vi "Lab Panel V6.00.vi"() -> ()   [LabVIEW 2017] (continued)
                    n3246 = call "sub vi-open serial port v1.vi"("Select COM port"=w5964) -> ("Error"=w5963:bool, "LOOPS"=w5962:i32, "VISA Com out"=w5961:refnum<visa-resource-name>)  [unwired: 12 in]
                    n3247 = local write "Com setup loops"(w5962) -> ()
                    n3248 = local write "Com Port Status"(w5963) -> ()
                    n3249 = local write "VISA Com out"(w5961) -> ()
                    n3250 = global write "Global 1.vi" "COM port"(w5961) -> ()
                  }
                }
              }
              frame #1 {
                # "only get temperature from initial valid temperature circuits, circuits detected at startup time"
                n3251 = local read "VISA Com out"() -> (w5974:refnum<visa-resource-name>)
                n3252 = global write "Global 1.vi" "COM port"(w5974) -> ()
                n3253 = local read "Temp read loop"() -> (w5971:dbl)
                n3254 = global write "Global 1.vi" "tmp dly lps"("Temp Delay Lps") -> ()
                n3255 = global write "Global 1.vi" "dly value"("Temp Value") -> ()
                n3256 = local read "jig cycle"() -> (w5975:dbl)
                n3257 = local read "on loops"() -> (w5977:dbl)
                n3258 = Equal?(x=w5971, y=1) -> (x = y?=w5968:bool)
                n3259 = Add(x=w5977, y=6) -> (x+y=w5978:dbl)
                n3260 = Equal?(x=w5975, y=w5978) -> (x = y?=w5969:bool)
                n3261 = And(x=w5969, y=w5968) -> (x .and. y?=w5967:bool)
                n3262 = Or(x=w5967, y="Read Temp") -> (x .or. y?=w5966:bool)
                n3263 = case shown="True" w5966 {
                  frame False {
                  }
                  frame True {
                    w5979 = TRUE
                    n3264 = local write "TEMP"(w5979) -> ()
                    n3265 = local write "Read Temp"(FALSE) -> ()
                    n3266 = stacked-sequence {
                      tunnel: 1.0 -> [_ _ _ _ w6012]
                      tunnel: "Temp Simulate" -> [_ _ _ _ w6011]
                      tunnel: w5979 -> [_ _ _ _ _]
                      frame #0 {
                        # "only switch relay on to reset temp circuits if busy testing"
                        n3267 = disable-structure shown="Enabled" {
                          frame Disabled {
                            n3268 = local read "Any Test Running"() -> ()  [unwired: 1 out]
                          }
                          frame Enabled {
                          }
                        }
                        n3269 = local read "USB OUT 0"() -> (w5984:bool[])
                        n3270 = local read "USB OUT 2"() -> (w5986:bool[])
                        n3271 = local read "USB OUT 1"() -> (w5985:bool[])
                        n3272 = Insert Into Array(array=w5986, index=7, new element=TRUE) -> (w5987:bool[])
                        n3273 = call "sub vi - Drive Relays All v6.vi"("Array #2"=w5987, "Array #1"=w5985, "Array #0"=w5984) -> ()  [unwired: 8 in, 1 out]
                      }
                      frame #1 {
                        # "time delay"
                        n3274 = Wait (ms)(milliseconds to wait=500) -> ()  [unwired: 1 out]
                      }
                      frame #2 {
                        # "switch relay off"
                        n3275 = local read "USB OUT 0"() -> (w5990:bool[])
                        n3276 = local read "USB OUT 2"() -> (w5992:bool[])
                        n3277 = local read "USB OUT 1"() -> (w5991:bool[])
                        n3278 = Insert Into Array(array=w5992, index=7, new element=FALSE) -> (w5993:bool[])
                        n3279 = call "sub vi - Drive Relays All v6.vi"("Array #2"=w5993, "Array #1"=w5991, "Array #0"=w5990) -> ()  [unwired: 8 in, 1 out]
                      }
                      frame #3 {
                        # "time delay"
                        n3280 = Wait (ms)(milliseconds to wait=300) -> ()  [unwired: 1 out]
                      }
                      frame #4 {
                        # "read all valid temp circuits"
                        n3281 = local read "LAB01-TP"() -> (w6004:bool)
                        n3282 = local read "LAB03-TP"() -> (w6002:bool)
                        n3283 = local read "LAB02-TP"() -> (w6003:bool)
                        n3284 = local read "LAB04-TP"() -> (w6001:bool)
                        n3285 = local read "LAB05-TP"() -> (w6005:bool)
                        n3286 = call "sub vi - GET ALL TEMP v7.vi"("LA01-EN"=w6004, "LA02-EN"=w6003, "LA03-EN"=w6002, "LA04-EN"=w6001, "LA05-EN"=w6005, "simulate"=w6011, "Gen Cal Value"=w6012) -> ("LOOP TIME"=→"Read Time":dbl, "Fault Counters"=→"Fault Counters":u64[], "error 1"=→"Error Temp":bool, "LA01 TEMP"=w6010:T30, "LA02 TEMP"=w6009:T30, "LA04 TEMP"=w6007:T30, "LA03 TEMP"=w6008:T30, "Errors"=→"TempErrors":bool[], "LA05 TEMP"=w6006:T30)  [unwired: 3 in, 1 out]
                        n3287 = local write "LAB01 TEMP"(w6010) -> ()
                        n3288 = local write "LAB02 TEMP"(w6009) -> ()
                        n3289 = local write "LAB03 TEMP"(w6008) -> ()
                        n3290 = local write "LAB04 TEMP"(w6007) -> ()
                        n3291 = local write "LAB05 TEMP"(w6006) -> ()
                      }
                    }
                  }
                }
              }
              frame #2 {
                n3292 = case shown="True" w6013 {
                  tunnel: w6026 -> [_ w6039]
                  tunnel: w6025 -> [_ w6038]
                  tunnel: w6024 -> [_ w6037]
                  tunnel: w6023 -> [_ w6036]
                  tunnel: w6022 -> [_ w6035]
                  tunnel: w6021 -> [_ w6034]
                  tunnel: w6020 -> [_ w6033]
                  tunnel: w6019 -> [_ w6032]
                  tunnel: w6018 -> [_ w6031]
                  tunnel: w6017 -> [_ w6030]
                  tunnel: w6016 -> [_ w6029]
                  tunnel: w6015 -> [_ w6028]
                  tunnel: w6014 -> [_ w6027]
                  frame False {
                  }
                  frame True {
                    n3293 = stacked-sequence {
                      tunnel: w6039 -> [_ w6052 w6097 w6142 w6187 w6232 _]
                      tunnel: w6038 -> [_ w6051 w6096 w6141 w6186 w6231 _]
                      tunnel: w6037 -> [_ w6041 _ _ _ _ _]
                      tunnel: w6036 -> [_ w6046 w6095 w6140 w6185 w6230 _]
                      tunnel: w6035 -> [_ w6040 _ _ _ _ _]
                      tunnel: w6034 -> [_ _ w6086 _ _ _ _]
                      tunnel: w6033 -> [_ _ w6085 _ _ _ _]
                      tunnel: w6032 -> [_ _ _ w6131 _ _ _]
                      tunnel: w6031 -> [_ _ _ w6130 _ _ _]
                      tunnel: w6030 -> [_ _ _ _ w6176 _ _]
                      tunnel: w6029 -> [_ _ _ _ w6175 _ _]
                      tunnel: w6028 -> [_ _ _ _ _ w6221 _]
                      tunnel: w6027 -> [_ _ _ _ _ w6220 _]
                      frame #0 {
                      }
                      frame #1 {
                        n3294 = case shown="False" w6052 {
                          tunnel: [w6083 w6084] -> w6068
                          tunnel: w6051 -> [_ w6084]
                          frame False {
                            n3295 = local read "CAL LAB01"() -> (w6083:T15)
                          }
                          frame True {
                          }
                        }
                        n3296 = local read "TEMP LA01"() -> (w6059:T9)
                        n3297 = local read "LAB01 TEMP"() -> (w6058:T12)
                        n3298 = call "sub vi - temperature delay v4.vi"("2-run"=w6040, "1-run"=w6041, "temp values IN"=w6059, "temp signals"=w6058) -> ("T2-N"=w6054:dbl, "T2-L"=w6055:dbl, "T1-N"=w6056:dbl, "T1-L"=w6057:dbl, "temp values OUT"=w6053:T51)  [unwired: 3 in]
                        n3299 = Unbundle By Name(w6068) -> ("1 (TL) cal"=w6063:dbl, "1 (TN) cal"=w6062:dbl, "2 (TL) cal"=w6061:dbl, "2 (TN) cal"=w6060:dbl)  [unwired: 6 out]
                        n3300 = local write "TEMP LA01"(w6053) -> ()
                        n3301 = Multiply(x=w6057, y=w6063) -> (x*y=w6050:dbl)
                        n3302 = Multiply(x=w6056, y=w6062) -> (x*y=w6048:dbl)
                        n3303 = Multiply(x=w6055, y=w6061) -> (x*y=w6045:dbl)
                        n3304 = Multiply(x=w6054, y=w6060) -> (x*y=w6044:dbl)
                        n3305 = case shown="True" w6041 {
                          tunnel: w6050 -> [w6077 w6082]
                          tunnel: w6046 -> [_ w6080]
                          tunnel: [w6077 w6081] -> w6049
                          tunnel: w6048 -> [w6076 w6079]
                          tunnel: [w6076 w6078] -> w6047
                          frame False {
                          }
                          frame True {
                            n3306 = Multiply(x=w6080, y=w6079) -> (x*y=w6078:dbl)
                            n3307 = Multiply(x=w6080, y=w6082) -> (x*y=w6081:dbl)
                          }
                        }
                        n3308 = case shown="True" w6040 {
                          tunnel: w6045 -> [w6070 w6075]
                          tunnel: w6046 -> [_ w6073]
                          tunnel: [w6070 w6074] -> w6043
                          tunnel: w6044 -> [w6069 w6072]
                          tunnel: [w6069 w6071] -> w6042
                          frame False {
                          }
                          frame True {
                            n3309 = Multiply(x=w6073, y=w6072) -> (x*y=w6071:dbl)
                            n3310 = Multiply(x=w6073, y=w6075) -> (x*y=w6074:dbl)
                          }
                        }
                        n3311 = local read "SIG LAB01-2"() -> (w6065:T2)
                        n3312 = local read "SIG LAB01-1"() -> (w6067:T2)
                        n3313 = Bundle By Name(cluster=w6067, "Tmp Live"=w6049, "Tmp Neut"=w6047) -> (w6066:T2)
                        n3314 = Bundle By Name(cluster=w6065, "Tmp Live"=w6043, "Tmp Neut"=w6042) -> (w6064:T2)
                        n3315 = local write "SIG LAB01-1"(w6066) -> ()
                        n3316 = local write "SIG LAB01-2"(w6064) -> ()
                      }
                      frame #2 {
                        n3317 = case shown="True" w6097 {
                          tunnel: [w6128 w6129] -> w6113
                          tunnel: w6096 -> [_ w6129]
                          frame False {
                            n3318 = local read "CAL LAB02"() -> (w6128:T16)
                          }
                          frame True {
                          }
                        }
                        n3319 = local read "LAB02 TEMP"() -> (w6104:T12)
                        n3320 = local read "TEMP LA02"() -> (w6103:T9)
                        n3321 = call "sub vi - temperature delay v4.vi"("2-run"=w6085, "1-run"=w6086, "temp values IN"=w6103, "temp signals"=w6104) -> ("T2-N"=w6098:dbl, "T2-L"=w6099:dbl, "T1-N"=w6100:dbl, "T1-L"=w6101:dbl, "temp values OUT"=w6102:T51)  [unwired: 3 in]
                        n3322 = Unbundle By Name(w6113) -> ("1 (TL) cal"=w6108:dbl, "1 (TN) cal"=w6107:dbl, "2 (TL) cal"=w6106:dbl, "2 (TN) cal"=w6105:dbl)  [unwired: 6 out]
                        n3323 = local write "TEMP LA02"(w6102) -> ()
                        n3324 = Multiply(x=w6101, y=w6108) -> (x*y=w6094:dbl)
                        n3325 = Multiply(x=w6100, y=w6107) -> (x*y=w6093:dbl)
                        n3326 = Multiply(x=w6099, y=w6106) -> (x*y=w6090:dbl)
                        n3327 = Multiply(x=w6098, y=w6105) -> (x*y=w6089:dbl)
                        n3328 = case shown="True" w6086 {
                          tunnel: w6094 -> [w6122 w6127]
                          tunnel: w6095 -> [_ w6125]
                          tunnel: [w6122 w6126] -> w6092
                          tunnel: w6093 -> [w6121 w6124]
                          tunnel: [w6121 w6123] -> w6091
                          frame False {
                          }
                          frame True {
                            n3329 = Multiply(x=w6125, y=w6124) -> (x*y=w6123:dbl)
                            n3330 = Multiply(x=w6125, y=w6127) -> (x*y=w6126:dbl)
                          }
                        }
                        n3331 = case shown="True" w6085 {
                          tunnel: w6090 -> [w6115 w6120]
                          tunnel: w6095 -> [_ w6118]
                          tunnel: [w6115 w6119] -> w6088
                          tunnel: w6089 -> [w6114 w6117]
                          tunnel: [w6114 w6116] -> w6087
                          frame False {
                          }
                          frame True {
                            n3332 = Multiply(x=w6118, y=w6117) -> (x*y=w6116:dbl)
                            n3333 = Multiply(x=w6118, y=w6120) -> (x*y=w6119:dbl)
                          }
                        }
                        n3334 = local read "SIG LAB02-2"() -> (w6110:T2)
                        n3335 = local read "SIG LAB02-1"() -> (w6112:T2)
                        n3336 = Bundle By Name(cluster=w6110, "Tmp Live"=w6088, "Tmp Neut"=w6087) -> (w6109:T2)
                        n3337 = Bundle By Name(cluster=w6112, "Tmp Live"=w6092, "Tmp Neut"=w6091) -> (w6111:T2)
                        n3338 = local write "SIG LAB02-1"(w6111) -> ()
                        n3339 = local write "SIG LAB02-2"(w6109) -> ()
                      }
                      frame #3 {
                        n3340 = case shown="False" w6142 {
                          tunnel: [w6173 w6174] -> w6158
                          tunnel: w6141 -> [_ w6174]
                          frame False {
                            n3341 = local read "CAL LAB03"() -> (w6173:T15)
                          }
                          frame True {
                          }
                        }
                        n3342 = local read "TEMP LA03"() -> (w6148:T9)
                        n3343 = local read "LAB03 TEMP"() -> (w6149:T12)
                        n3344 = call "sub vi - temperature delay v4.vi"("2-run"=w6130, "1-run"=w6131, "temp values IN"=w6148, "temp signals"=w6149) -> ("T2-N"=w6143:dbl, "T2-L"=w6144:dbl, "T1-N"=w6145:dbl, "T1-L"=w6146:dbl, "temp values OUT"=w6147:T51)  [unwired: 3 in]
                        n3345 = Unbundle By Name(w6158) -> ("1 (TL) cal"=w6153:dbl, "1 (TN) cal"=w6152:dbl, "2 (TL) cal"=w6151:dbl, "2 (TN) cal"=w6150:dbl)  [unwired: 6 out]
                        n3346 = local write "TEMP LA03"(w6147) -> ()
                        n3347 = Multiply(x=w6146, y=w6153) -> (x*y=w6139:dbl)
                        n3348 = Multiply(x=w6145, y=w6152) -> (x*y=w6138:dbl)
                        n3349 = Multiply(x=w6144, y=w6151) -> (x*y=w6135:dbl)
                        n3350 = Multiply(x=w6143, y=w6150) -> (x*y=w6134:dbl)
                        n3351 = case shown="True" w6130 {
                          tunnel: w6135 -> [w6160 w6165]
                          tunnel: w6140 -> [_ w6163]
                          tunnel: [w6160 w6164] -> w6133
                          tunnel: w6134 -> [w6159 w6162]
                          tunnel: [w6159 w6161] -> w6132
                          frame False {
                          }
                          frame True {
                            n3352 = Multiply(x=w6163, y=w6162) -> (x*y=w6161:dbl)
                            n3353 = Multiply(x=w6163, y=w6165) -> (x*y=w6164:dbl)
                          }
                        }
                        n3354 = case shown="True" w6131 {
                          tunnel: w6139 -> [w6167 w6172]
                          tunnel: w6140 -> [_ w6170]
                          tunnel: [w6167 w6171] -> w6137
                          tunnel: w6138 -> [w6166 w6169]
                          tunnel: [w6166 w6168] -> w6136
                          frame False {
                          }
                          frame True {
                            n3355 = Multiply(x=w6170, y=w6169) -> (x*y=w6168:dbl)
                            n3356 = Multiply(x=w6170, y=w6172) -> (x*y=w6171:dbl)
                          }
                        }
                        n3357 = local read "SIG LAB03-2"() -> (w6155:T2)
                        n3358 = local read "SIG LAB03-1"() -> (w6157:T2)
                        n3359 = Bundle By Name(cluster=w6155, "Tmp Live"=w6133, "Tmp Neut"=w6132) -> (w6154:T2)
                        n3360 = Bundle By Name(cluster=w6157, "Tmp Live"=w6137, "Tmp Neut"=w6136) -> (w6156:T2)
                        n3361 = local write "SIG LAB03-2"(w6154) -> ()
                        n3362 = local write "SIG LAB03-1"(w6156) -> ()
                      }
                      frame #4 {
                        n3363 = case shown="False" w6187 {
                          tunnel: [w6218 w6219] -> w6203
                          tunnel: w6186 -> [_ w6219]
                          frame False {
                            n3364 = local read "CAL LAB04"() -> (w6218:T15)
                          }
                          frame True {
                          }
                        }
                        n3365 = local read "LAB04 TEMP"() -> (w6193:T12)
                        n3366 = local read "TEMP LA04"() -> (w6194:T9)
                        n3367 = call "sub vi - temperature delay v4.vi"("2-run"=w6175, "1-run"=w6176, "temp values IN"=w6194, "temp signals"=w6193) -> ("T2-N"=w6188:dbl, "T2-L"=w6189:dbl, "T1-N"=w6190:dbl, "T1-L"=w6191:dbl, "temp values OUT"=w6192:T51)  [unwired: 3 in]
                        n3368 = Unbundle By Name(w6203) -> ("1 (TL) cal"=w6198:dbl, "1 (TN) cal"=w6197:dbl, "2 (TL) cal"=w6196:dbl, "2 (TN) cal"=w6195:dbl)  [unwired: 6 out]
                        n3369 = local write "TEMP LA04"(w6192) -> ()
                        n3370 = Multiply(x=w6191, y=w6198) -> (x*y=w6184:dbl)
                        n3371 = Multiply(x=w6190, y=w6197) -> (x*y=w6183:dbl)
                        n3372 = Multiply(x=w6189, y=w6196) -> (x*y=w6180:dbl)
                        n3373 = Multiply(x=w6188, y=w6195) -> (x*y=w6179:dbl)
                        n3374 = case shown="True" w6175 {
                          tunnel: w6180 -> [w6205 w6210]
                          tunnel: w6185 -> [_ w6208]
                          tunnel: [w6205 w6209] -> w6178
                          tunnel: w6179 -> [w6204 w6207]
                          tunnel: [w6204 w6206] -> w6177
                          frame False {
                          }
                          frame True {
                            n3375 = Multiply(x=w6208, y=w6207) -> (x*y=w6206:dbl)
                            n3376 = Multiply(x=w6208, y=w6210) -> (x*y=w6209:dbl)
                          }
                        }
                        n3377 = case shown="True" w6176 {
                          tunnel: w6184 -> [w6212 w6217]
                          tunnel: w6185 -> [_ w6215]
                          tunnel: [w6212 w6216] -> w6182
                          tunnel: w6183 -> [w6211 w6214]
                          tunnel: [w6211 w6213] -> w6181
                          frame False {
                          }
                          frame True {
                            n3378 = Multiply(x=w6215, y=w6214) -> (x*y=w6213:dbl)
                            n3379 = Multiply(x=w6215, y=w6217) -> (x*y=w6216:dbl)
                          }
                        }
                        n3380 = local read "SIG LAB04-2"() -> (w6200:T2)
                        n3381 = local read "SIG LAB04-1"() -> (w6202:T2)
                        n3382 = Bundle By Name(cluster=w6200, "Tmp Live"=w6178, "Tmp Neut"=w6177) -> (w6199:T2)
                        n3383 = Bundle By Name(cluster=w6202, "Tmp Live"=w6182, "Tmp Neut"=w6181) -> (w6201:T2)
                        n3384 = local write "SIG LAB04-2"(w6199) -> ()
                        n3385 = local write "SIG LAB04-1"(w6201) -> ()
                      }
                      frame #5 {
                        n3386 = case shown="True" w6232 {
                          tunnel: [w6263 T15 {"1  (A) cal"=1.0, "1 (V) cal"=1.0, "1 (PF) cal"=1.0, "1 (TL) cal"=1.0, "1 (TN) cal"=1.0, "2 (A) cal"=1.0, "2 (V) cal"=1.0, "2 (PF) cal"=1.0, "2 (TL) cal"=1.0, "2 (TN) cal"=1.0} ("LAB05 (CAL) 2")] -> w6248
                          tunnel: w6231 -> [_ _]
                          frame False {
                            n3387 = local read "LAB05 (CAL)"() -> (w6263:T15)
                          }
                          frame True {
                          }
                        }
                        n3388 = local read "LAB05 TEMP"() -> (w6238:T12)
                        n3389 = local read "TEMP LA05"() -> (w6239:T9)
                        n3390 = call "sub vi - temperature delay v4.vi"("2-run"=w6220, "1-run"=w6221, "temp values IN"=w6239, "temp signals"=w6238) -> ("T2-N"=w6234:dbl, "T2-L"=w6235:dbl, "T1-N"=w6236:dbl, "T1-L"=w6237:dbl, "temp values OUT"=w6233:T51)  [unwired: 3 in]
                        n3391 = local write "TEMP LA05"(w6233) -> ()
                        n3392 = Unbundle By Name(w6248) -> ("1 (TL) cal"=w6240:dbl, "1 (TN) cal"=w6243:dbl, "2 (TL) cal"=w6242:dbl, "2 (TN) cal"=w6241:dbl)  [unwired: 6 out]
                        n3393 = Multiply(x=w6237, y=w6240) -> (x*y=w6229:dbl)
                        n3394 = Multiply(x=w6236, y=w6243) -> (x*y=w6228:dbl)
                        n3395 = Multiply(x=w6235, y=w6242) -> (x*y=w6225:dbl)
                        n3396 = Multiply(x=w6234, y=w6241) -> (x*y=w6224:dbl)
                        n3397 = case shown="True" w6220 {
                          tunnel: w6225 -> [w6250 w6255]
                          tunnel: w6230 -> [_ w6253]
                          tunnel: [w6250 w6254] -> w6223
                          tunnel: w6224 -> [w6249 w6252]
                          tunnel: [w6249 w6251] -> w6222
                          frame False {
                          }
                          frame True {
                            n3398 = Multiply(x=w6253, y=w6252) -> (x*y=w6251:dbl)
                            n3399 = Multiply(x=w6253, y=w6255) -> (x*y=w6254:dbl)
                          }
                        }
                        n3400 = case shown="True" w6221 {
                          tunnel: w6229 -> [w6257 w6262]
                          tunnel: w6230 -> [_ w6260]
                          tunnel: [w6257 w6261] -> w6227
                          tunnel: w6228 -> [w6256 w6259]
                          tunnel: [w6256 w6258] -> w6226
                          frame False {
                          }
                          frame True {
                            n3401 = Multiply(x=w6260, y=w6259) -> (x*y=w6258:dbl)
                            n3402 = Multiply(x=w6260, y=w6262) -> (x*y=w6261:dbl)
                          }
                        }
                        n3403 = local read "SIG LAB05-1"() -> (w6247:T2)
                        n3404 = Bundle By Name(cluster=w6247, "Tmp Live"=w6227, "Tmp Neut"=w6226) -> (w6246:T2)
                        n3405 = local read "SIG LAB05-2"() -> (w6245:T2)
                        n3406 = Bundle By Name(cluster=w6245, "Tmp Live"=w6223, "Tmp Neut"=w6222) -> (w6244:T2)
                        n3407 = local write "SIG LAB05-1"(w6246) -> ()
                        n3408 = local write "SIG LAB05-2"(w6244) -> ()
                      }
                      frame #6 {
                        w6365 = 150.0
                        # "check for thermocouple error, output >150 deg??"
                        n3409 = local read "SIG LAB01-2"() -> (w6374:T2)
                        n3410 = local read "SIG LAB01-1"() -> (w6375:T2)
                        n3411 = local read "SIG LAB04-1"() -> (w6368:T2)
                        n3412 = local read "SIG LAB04-2"() -> (w6369:T2)
                        n3413 = Unbundle By Name(w6375) -> ("Tmp Live"=w6303:dbl, "Tmp Neut"=w6301:dbl)
                        n3414 = Unbundle(w6369) -> ("Tmp Live"=w6279:dbl, "Tmp Neut"=w6278:dbl)  [unwired: 3 out]
                        n3415 = Unbundle(w6374) -> ("Tmp Live"=w6300:dbl, "Tmp Neut"=w6298:dbl)  [unwired: 3 out]
                        n3416 = Unbundle(w6368) -> ("Tmp Live"=w6280:dbl, "Tmp Neut"=w6273:dbl)  [unwired: 3 out]
                        n3417 = Absolute Value(x=w6280) -> (abs(x)=w6274:dbl)
                        n3418 = Absolute Value(x=w6273) -> (abs(x)=w6275:dbl)
                        n3419 = Absolute Value(x=w6279) -> (abs(x)=w6277:dbl)
                        n3420 = Absolute Value(x=w6278) -> (abs(x)=w6276:dbl)
                        n3421 = Absolute Value(x=w6300) -> (abs(x)=w6299:dbl)
                        n3422 = Absolute Value(x=w6298) -> (abs(x)=w6297:dbl)
                        n3423 = Absolute Value(x=w6301) -> (abs(x)=w6302:dbl)
                        n3424 = Absolute Value(x=w6303) -> (abs(x)=w6304:dbl)
                        n3425 = Greater?(x=w6276, y=w6365) -> (0:w6341:bool)
                        "LA04-2 (TN)" <- w6341
                        n3426 = Greater?(x=w6297, y=w6365) -> (0:w6353:bool)
                        "LA01-2 (TN)" <- w6353
                        n3427 = Greater?(x=w6277, y=w6365) -> (0:w6342:bool)
                        "LA04-2 (TL)" <- w6342
                        n3428 = Greater?(x=w6299, y=w6365) -> (0:w6354:bool)
                        "LA01-2 (TL)" <- w6354
                        n3429 = Greater?(x=w6275, y=w6365) -> (0:w6343:bool)
                        "LA04-1 (TN)" <- w6343
                        n3430 = Greater?(x=w6302, y=w6365) -> (0:w6364:bool)
                        "LA01-1 (TN)" <- w6364
                        n3431 = Greater?(x=w6274, y=w6365) -> (0:w6344:bool)
                        "LA04-1 (TL)" <- w6344
                        n3432 = Greater?(x=w6304, y=w6365) -> (0:w6363:bool)
                        "LA01-1 (TL)" <- w6363
                        n3433 = Or(x=w6364, y=w6363) -> (x .or. y?=w6362:bool)
                        n3434 = Or(x=w6341, y=w6342) -> (x .or. y?=w6352:bool)
                        n3435 = Or(x=w6354, y=w6353) -> (x .or. y?=w6358:bool)
                        n3436 = Or(x=w6343, y=w6344) -> (x .or. y?=w6348:bool)
                        n3437 = Select(t=u32 16711680, s=w6362, f=u32 13816530) -> (s? t:f=w6359:u32)
                        n3438 = Select(t=u32 16711680, s=w6352, f=u32 13816530) -> (s? t:f=w6349:u32)
                        n3439 = Select(t=u32 16711680, s=w6358, f=u32 13816530) -> (s? t:f=w6355:u32)
                        n3440 = Select(t=u32 16711680, s=w6348, f=u32 13816530) -> (s? t:f=w6345:u32)
                        n3441 = property on="SIG LAB01-1" class="Clust (strict)"("Color"=w6359) -> ()  [unwired: 2 in, 2 out]
                        n3442 = property on="SIG LAB01-2" class="Clust (strict)"("Color"=w6355) -> ()  [unwired: 2 in, 2 out]
                        n3443 = property on="SIG LAB04-2" class="Clust (strict)"("Color"=w6349) -> ()  [unwired: 2 in, 2 out]
                        n3444 = property on="SIG LAB04-1" class="Clust (strict)"("Color"=w6345) -> ()  [unwired: 2 in, 2 out]
                        n3445 = local read "SIG LAB02-1"() -> (w6372:T2)
                        n3446 = local read "SIG LAB02-2"() -> (w6373:T2)
                        n3447 = local read "SIG LAB05-2"() -> (w6366:T2)
                        n3448 = local read "SIG LAB05-1"() -> (w6367:T2)
                        n3449 = Unbundle(w6373) -> ("Tmp Live"=w6292:dbl, "Tmp Neut"=w6290:dbl)  [unwired: 3 out]
                        n3450 = Unbundle(w6372) -> ("Tmp Live"=w6296:dbl, "Tmp Neut"=w6295:dbl)  [unwired: 3 out]
                        n3451 = Unbundle(w6366) -> ("Tmp Live"=w6268:dbl, "Tmp Neut"=w6266:dbl)  [unwired: 3 out]
                        n3452 = Unbundle(w6367) -> ("Tmp Live"=w6272:dbl, "Tmp Neut"=w6270:dbl)  [unwired: 3 out]
                        n3453 = Absolute Value(x=w6292) -> (abs(x)=w6291:dbl)
                        n3454 = Absolute Value(x=w6290) -> (abs(x)=w6289:dbl)
                        n3455 = Absolute Value(x=w6295) -> (abs(x)=w6293:dbl)
                        n3456 = Absolute Value(x=w6296) -> (abs(x)=w6294:dbl)
                        n3457 = Absolute Value(x=w6268) -> (abs(x)=w6267:dbl)
                        n3458 = Absolute Value(x=w6266) -> (abs(x)=w6265:dbl)
                        n3459 = Absolute Value(x=w6272) -> (abs(x)=w6271:dbl)
                        n3460 = Absolute Value(x=w6270) -> (abs(x)=w6269:dbl)
                        n3461 = Greater?(x=w6289, y=w6365) -> (0:w6317:bool)
                        "LA02-2 (TN)" <- w6317
                        n3462 = Greater?(x=w6291, y=w6365) -> (0:w6318:bool)
                        "LA02-2 (TL)" <- w6318
                        n3463 = Greater?(x=w6293, y=w6365) -> (0:w6320:bool)
                        "LA02-1 (TN)" <- w6320
                        n3464 = Greater?(x=w6294, y=w6365) -> (0:w6319:bool)
                        "LA02-1 (TL)" <- w6319
                        n3465 = Greater?(x=w6265, y=w6365) -> (0:w6329:bool)
                        "LA05-2 (TN)" <- w6329
                        n3466 = Greater?(x=w6267, y=w6365) -> (0:w6330:bool)
                        "LA05-2 (TL)" <- w6330
                        n3467 = Greater?(x=w6269, y=w6365) -> (0:w6331:bool)
                        "LA05-1 (TN)" <- w6331
                        n3468 = Greater?(x=w6271, y=w6365) -> (0:w6332:bool)
                        "LA05-1 (TL)" <- w6332
                        n3469 = Or(x=w6320, y=w6319) -> (x .or. y?=w6328:bool)
                        n3470 = Or(x=w6318, y=w6317) -> (x .or. y?=w6324:bool)
                        n3471 = Or(x=w6332, y=w6331) -> (x .or. y?=w6340:bool)
                        n3472 = Or(x=w6330, y=w6329) -> (x .or. y?=w6336:bool)
                        n3473 = Select(t=u32 16711680, s=w6328, f=u32 13816530) -> (s? t:f=w6325:u32)
                        n3474 = Select(t=u32 16711680, s=w6324, f=u32 13816530) -> (s? t:f=w6321:u32)
                        n3475 = Select(t=u32 16711680, s=w6340, f=u32 13816530) -> (s? t:f=w6337:u32)
                        n3476 = local read "SIG LAB03-1"() -> (w6370:T2)
                        n3477 = Select(t=u32 16711680, s=w6336, f=u32 13816530) -> (s? t:f=w6333:u32)
                        n3478 = property on="SIG LAB02-1" class="Clust (strict)"("Color"=w6325) -> ()  [unwired: 2 in, 2 out]
                        n3479 = property on="SIG LAB02-2" class="Clust (strict)"("Color"=w6321) -> ()  [unwired: 2 in, 2 out]
                        n3480 = local read "SIG LAB03-2"() -> (w6371:T2)
                        n3481 = property on="SIG LAB05-1" class="Clust (strict)"("Color"=w6337) -> ()  [unwired: 2 in, 2 out]
                        n3482 = property on="SIG LAB05-2" class="Clust (strict)"("Color"=w6333) -> ()  [unwired: 2 in, 2 out]
                        n3483 = Unbundle(w6371) -> ("Tmp Live"=w6284:dbl, "Tmp Neut"=w6282:dbl)  [unwired: 3 out]
                        n3484 = Unbundle(w6370) -> ("Tmp Live"=w6288:dbl, "Tmp Neut"=w6286:dbl)  [unwired: 3 out]
                        n3485 = Absolute Value(x=w6284) -> (abs(x)=w6283:dbl)
                        n3486 = Absolute Value(x=w6282) -> (abs(x)=w6281:dbl)
                        n3487 = Absolute Value(x=w6288) -> (abs(x)=w6287:dbl)
                        n3488 = Absolute Value(x=w6286) -> (abs(x)=w6285:dbl)
                        n3489 = Greater?(x=w6281, y=w6365) -> (0:w6305:bool)
                        "LA03-2 (TN)" <- w6305
                        n3490 = Greater?(x=w6283, y=w6365) -> (0:w6306:bool)
                        "LA03-2 (TL)" <- w6306
                        n3491 = Greater?(x=w6285, y=w6365) -> (0:w6308:bool)
                        "LA03-1 (TN)" <- w6308
                        n3492 = Greater?(x=w6287, y=w6365) -> (0:w6307:bool)
                        "LA03-1 (TL)" <- w6307
                        n3493 = Or(x=w6308, y=w6307) -> (x .or. y?=w6316:bool)
                        n3494 = Or(x=w6306, y=w6305) -> (x .or. y?=w6312:bool)
                        n3495 = Select(t=u32 16711680, s=w6316, f=u32 13816530) -> (s? t:f=w6313:u32)
                        n3496 = Select(t=u32 16711680, s=w6312, f=u32 13816530) -> (s? t:f=w6309:u32)
                        n3497 = property on="SIG LAB03-1" class="Clust (strict)"("Color"=w6313) -> ()  [unwired: 2 in, 2 out]
                        n3498 = property on="SIG LAB03-2" class="Clust (strict)"("Color"=w6309) -> ()  [unwired: 2 in, 2 out]
                      }
                    }
                  }
                }
              }
            }
          }
          frame #22 {
            # "SAVE ON AMPS VALUES FOR REPORT FILE"
            # "write data to display panel"
            n3499 = global write "Global display 1.vi" "TEST 5-2"(w6411) -> ()
            n3500 = global write "Global display 1.vi" "TEST 4-2"(w6413) -> ()
            n3501 = global write "Global display 1.vi" "TEST 1-2"(w6419) -> ()
            n3502 = global write "Global display 1.vi" "TEST 3-1"(w6416) -> ()
            n3503 = global write "Global display 1.vi" "TEST 5-1"(w6412) -> ()
            n3504 = global write "Global display 1.vi" "TEST 1-1"(w6420) -> ()
            n3505 = global write "Global display 1.vi" "TEST 3-2"(w6415) -> ()
            n3506 = global write "Global display 1.vi" "TEST 4-1"(w6414) -> ()
            n3507 = global write "Global display 1.vi" "TEST 2-2"(w6417) -> ()
            n3508 = global write "Global display 1.vi" "TEST 2-1"(w6418) -> ()
            n3509 = global read "Global display 3.vi" "log 1-1"() -> (→"LOG LAB01-1":string)
            n3510 = global read "Global display 3.vi" "log 3-1"() -> (→"LOG LAB03-1":string)
            n3511 = global read "Global display 3.vi" "log 1-2"() -> (→"LOG LAB01-2":string)
            n3512 = property on="Tab Control 2" class="TabCtl (strict)"() -> ("Pages"=w6410:refnum<vi>[])  [unwired: 2 in, 2 out]
            n3513 = global read "Global display 3.vi" "log 2-1"() -> (→"LOG LAB02-1":string)
            n3514 = global read "Global display 3.vi" "log 2-2"() -> (→"LOG LAB02-2":string)
            n3515 = global read "Global display 3.vi" "log 4-2"() -> (→"LOG LAB04-2":string)
            n3516 = global read "Global display 3.vi" "log 5-2"() -> (→"LOG LAB05-2":string)
            n3517 = global read "Global display 3.vi" "log 5-1"() -> (→"LOG LAB05-1":string)
            n3518 = global read "Global display 3.vi" "log 4-1"() -> (→"LOG LAB04-1":string)
            n3519 = global read "Global display 3.vi" "log 3-2"() -> (→"LOG LAB03-2":string)
            n3520 = Index Array(array=w6410, index=8) -> (element=w6408:refnum<vi>)
            n3521 = property class="Page"(reference=w6408) -> ("PageVis"=w6407:bool)  [unwired: 1 in, 2 out]
            n3522 = local read "DISP LAB03-1"() -> (w6446:T4)
            n3523 = local read "DISP LAB04-2"() -> (w6443:T4)
            n3524 = local read "DISP LAB05-1"() -> (w6442:T4)
            n3525 = local read "DISP LAB01-2"() -> (w6449:T4)
            n3526 = local read "DISP LAB02-1"() -> (w6448:T4)
            n3527 = local read "DISP LAB02-2"() -> (w6447:T4)
            n3528 = local read "DISP LAB04-1"() -> (w6444:T4)
            n3529 = local read "DISP LAB05-2"() -> (w6441:T4)
            n3530 = local read "DISP LAB01-1"() -> (w6450:T4)
            n3531 = local read "DISP LAB03-2"() -> (w6445:T4)
            n3532 = global write "Global display 3.vi" "admin"(w6407) -> ()
            n3533 = local read "O/I  LAB05-2"() -> (w6461:bool)
            n3534 = local read "O/I  LAB05-1"() -> (w6462:bool)
            n3535 = local read "O/I  LAB03-2"() -> (w6465:bool)
            n3536 = local read "O/I  LAB04-2"() -> (w6463:bool)
            n3537 = local read "O/I  LAB04-1"() -> (w6464:bool)
            n3538 = local read "O/I  LAB03-1"() -> (w6466:bool)
            n3539 = local read "O/I  LAB01-2"() -> (w6469:bool)
            n3540 = local read "O/I  LAB01-1"() -> (w6470:bool)
            n3541 = local read "O/I  LAB02-1"() -> (w6468:bool)
            n3542 = local read "O/I  LAB02-2"() -> (w6467:bool)
            n3543 = global write "Global display 1.vi" "5-2 O/F"(w6461) -> ()
            n3544 = global write "Global display 1.vi" "5-1 O/F"(w6462) -> ()
            n3545 = global write "Global display 1.vi" "4-1 O/F"(w6464) -> ()
            n3546 = global write "Global display 1.vi" "4-2 O/F"(w6463) -> ()
            n3547 = global write "Global display 2.vi" "DISP LAB02-1"(w6448) -> ()
            n3548 = global write "Global display 2.vi" "DISP LAB02-2"(w6447) -> ()
            n3549 = global write "Global display 2.vi" "DISP LAB05-1"(w6442) -> ()
            n3550 = global write "Global display 2.vi" "DISP LAB05-2"(w6441) -> ()
            n3551 = global write "Global display 1.vi" "3-2 O/F"(w6465) -> ()
            n3552 = global write "Global display 2.vi" "DISP LAB01-2"(w6449) -> ()
            n3553 = global write "Global display 2.vi" "DISP LAB04-2"(w6443) -> ()
            n3554 = global write "Global display 2.vi" "DISP LAB01-1"(w6450) -> ()
            n3555 = global write "Global display 2.vi" "DISP LAB03-1"(w6446) -> ()
            n3556 = global write "Global display 1.vi" "3-1 O/F"(w6466) -> ()
            n3557 = global write "Global display 2.vi" "DISP LAB04-1"(w6444) -> ()
            n3558 = global write "Global display 1.vi" "2-2 O/F"(w6467) -> ()
            n3559 = global write "Global display 2.vi" "DISP LAB03-2"(w6445) -> ()
            n3560 = global write "Global display 1.vi" "2-1 O/F"(w6468) -> ()
            n3561 = global write "Global display 1.vi" "1-2 O/F"(w6469) -> ()
            n3562 = global write "Global display 1.vi" "1-1 O/F"(w6470) -> ()
            n3563 = local read "run lab05-2"() -> (w6451:bool)
            n3564 = local read "run lab04-1"() -> (w6454:bool)
            n3565 = local read "run lab04-2"() -> (w6453:bool)
            n3566 = local read "run lab05-1"() -> (w6452:bool)
            n3567 = local read "TEMP START LAB02-2"() -> (w6393:cluster{"TL":dbl, "TN":dbl})
            n3568 = local read "TEMP START LAB01-2"() -> (w6395:cluster{"TL":dbl, "TN":dbl})
            n3569 = local read "TEMP START LAB02-1"() -> (w6394:cluster{"TL":dbl, "TN":dbl})
            n3570 = local read "TEMP START LAB04-1"() -> (w6390:cluster{"TL":dbl, "TN":dbl})
            n3571 = local read "TEMP START LAB04-2"() -> (w6389:cluster{"TL":dbl, "TN":dbl})
            n3572 = local read "run lab03-2"() -> (w6455:bool)
            n3573 = local read "TEMP START LAB01-1"() -> (w6396:cluster{"TL":dbl, "TN":dbl})
            n3574 = local read "TEMP START LAB05-2"() -> (w6387:cluster{"TL":dbl, "TN":dbl})
            n3575 = local read "TEMP START LAB05-1"() -> (w6388:cluster{"TL":dbl, "TN":dbl})
            n3576 = local read "run lab02-1"() -> (w6458:bool)
            n3577 = local read "run lab03-1"() -> (w6456:bool)
            n3578 = local read "TEMP START LAB03-2"() -> (w6391:cluster{"TL":dbl, "TN":dbl})
            n3579 = local read "run lab01-2"() -> (w6459:bool)
            n3580 = local read "run lab02-2"() -> (w6457:bool)
            n3581 = local read "TEMP START LAB03-1"() -> (w6392:cluster{"TL":dbl, "TN":dbl})
            n3582 = local read "run lab01-1"() -> (w6460:bool)
            n3583 = global write "Global display 1.vi" "5-2 R/S"(w6451) -> ()
            n3584 = global write "Global display 1.vi" "5-1 R/S"(w6452) -> ()
            n3585 = global write "Global display 1.vi" "4-2 R/S"(w6453) -> ()
            n3586 = global write "Global display 1.vi" "4-1 R/S"(w6454) -> ()
            n3587 = global write "Global display 1.vi" "3-2 R/S"(w6455) -> ()
            n3588 = global write "Global display 1.vi" "1-2 R/S"(w6459) -> ()
            n3589 = global write "Global display 1.vi" "2-1 R/S"(w6458) -> ()
            n3590 = global write "Global display 1.vi" "3-1 R/S"(w6456) -> ()
            n3591 = global write "Global display 1.vi" "2-2 R/S"(w6457) -> ()
            n3592 = global write "Global display 1.vi" "1-1 R/S"(w6460) -> ()
            n3593 = local read "SET LAB05-2"() -> (w6431:T5)
            n3594 = local read "SET LAB05-1"() -> (w6432:T5)
            n3595 = local read "SET LAB04-1"() -> (w6434:T5)
            n3596 = local read "SET LAB04-2"() -> (w6433:T5)
            n3597 = local read "SET LAB01-1"() -> (w6440:T5)
            n3598 = local read "SET LAB03-1"() -> (w6436:T5)
            n3599 = local read "SET LAB03-2"() -> (w6435:T5)
            n3600 = local read "SET LAB02-2"() -> (w6437:T5)
            n3601 = local read "SET LAB01-2"() -> (w6439:T5)
            n3602 = local read "SET LAB02-1"() -> (w6438:T5)
            n3603 = global write "Global display 3.vi" "TEMP ST 05-2"(w6387) -> ()
            n3604 = global write "Global display 3.vi" "TEMP ST 05-1"(w6388) -> ()
            n3605 = global write "Global display 3.vi" "TEMP ST 03-2"(w6391) -> ()
            n3606 = global write "Global display 3.vi" "TEMP ST 04-2"(w6389) -> ()
            n3607 = global write "Global display 3.vi" "TEMP ST 01-1"(w6396) -> ()
            n3608 = global write "Global display 3.vi" "TEMP ST 01-2"(w6395) -> ()
            n3609 = global write "Global display 3.vi" "TEMP ST 04-1"(w6390) -> ()
            n3610 = global write "Global display 3.vi" "TEMP ST 02-1"(w6394) -> ()
            n3611 = global write "Global display 3.vi" "TEMP ST 02-2"(w6393) -> ()
            n3612 = global write "Global display 3.vi" "TEMP ST 03-1"(w6392) -> ()
            n3613 = global write "Global display 2.vi" "SET LAB05-2"(w6431) -> ()
            n3614 = global write "Global display 2.vi" "SET LAB05-1"(w6432) -> ()
            n3615 = global write "Global display 2.vi" "SET LAB04-1"(w6434) -> ()
            n3616 = global write "Global display 2.vi" "SET LAB01-1"(w6440) -> ()
            n3617 = global write "Global display 2.vi" "SET LAB04-2"(w6433) -> ()
            n3618 = global write "Global display 2.vi" "SET LAB03-2"(w6435) -> ()
            n3619 = global write "Global display 2.vi" "SET LAB02-2"(w6437) -> ()
            n3620 = global write "Global display 2.vi" "SET LAB03-1"(w6436) -> ()
            n3621 = global write "Global display 2.vi" "SET LAB01-2"(w6439) -> ()
            n3622 = global write "Global display 2.vi" "SET LAB02-1"(w6438) -> ()
            n3623 = local read "TEMP RISE LAB05-1"() -> (w6378:cluster{"TL":dbl, "TN":dbl})
            n3624 = local read "TEMP RISE LAB05-2"() -> (w6377:cluster{"TL":dbl, "TN":dbl})
            n3625 = local read "TEMP RISE LAB04-2"() -> (w6379:cluster{"TL":dbl, "TN":dbl})
            n3626 = local read "TEMP RISE LAB04-1"() -> (w6380:cluster{"TL":dbl, "TN":dbl})
            n3627 = local read "TEMP RISE LAB03-2"() -> (w6381:cluster{"TL":dbl, "TN":dbl})
            n3628 = local read "TEMP RISE LAB03-1"() -> (w6382:cluster{"TL":dbl, "TN":dbl})
            n3629 = local read "TEMP RISE LAB01-2"() -> (w6385:cluster{"TL":dbl, "TN":dbl})
            n3630 = local read "TEMP RISE LAB02-2"() -> (w6383:cluster{"TL":dbl, "TN":dbl})
            n3631 = local read "TEMP RISE LAB01-1"() -> (w6386:cluster{"TL":dbl, "TN":dbl})
            n3632 = local read "TEMP RISE LAB02-1"() -> (w6384:cluster{"TL":dbl, "TN":dbl})
            n3633 = local read "RESULT LAB01-1"() -> (w6430:bool)
            n3634 = local read "RESULT LAB03-2"() -> (w6425:bool)
            n3635 = local read "RESULT LAB04-1"() -> (w6424:bool)
            n3636 = local read "RESULT LAB04-2"() -> (w6423:bool)
            n3637 = local read "RESULT LAB02-2"() -> (w6427:bool)
            n3638 = local read "RESULT LAB01-2"() -> (w6429:bool)
            n3639 = local read "RESULT LAB02-1"() -> (w6428:bool)
            n3640 = local read "RESULT LAB03-1"() -> (w6426:bool)
            n3641 = local read "RESULT LAB05-1"() -> (w6422:bool)
            n3642 = local read "RESULT LAB05-2"() -> (w6421:bool)
            n3643 = local read "Amps Fail level"() -> (w6376:dbl)
            n3644 = stacked-sequence {
              tunnel: w6376 -> [w6472 w6477 w6482 w6487 w6492 w6497 w6502 w6507 w6512 w6517]
              frame #0 {
                n3645 = local read "SIG LAB01-1"() -> (w6474:T2)
                n3646 = Unbundle(w6474) -> ("AMPS"=w6473:dbl)  [unwired: 4 out]
                n3647 = Greater?(x=w6473, y=w6472) -> (0:w6471:bool)
                n3648 = case shown="True" w6471 {
                  frame False {
                  }
                  frame True {
                    n3649 = local read "ON L01-1"() -> (w6475:cluster{"amps":dbl, "volts":dbl, "pf":dbl})
                    n3650 = global write "Global display 2.vi" "ON L01-1"(w6475) -> ()
                  }
                }
              }
              frame #1 {
                n3651 = local read "SIG LAB01-2"() -> (w6479:T2)
                n3652 = Unbundle By Name(w6479) -> ("AMPS"=w6478:dbl)
                n3653 = Greater?(x=w6478, y=w6477) -> (0:w6476:bool)
                n3654 = case shown="True" w6476 {
                  frame False {
                  }
                  frame True {
                    n3655 = local read "ON L01-2"() -> (w6480:cluster{"amps":dbl, "volts":dbl, "pf":dbl})
                    n3656 = global write "Global display 2.vi" "ON L01-2"(w6480) -> ()
                  }
                }
              }
              frame #2 {
                n3657 = local read "SIG LAB02-1"() -> (w6484:T2)
                n3658 = Unbundle(w6484) -> ("AMPS"=w6483:dbl)  [unwired: 4 out]
                n3659 = Greater?(x=w6483, y=w6482) -> (0:w6481:bool)
                n3660 = case shown="True" w6481 {
                  frame False {
                  }
                  frame True {
                    n3661 = local read "ON L02-1"() -> (w6485:cluster{"amps":dbl, "volts":dbl, "pf":dbl})
                    n3662 = global write "Global display 2.vi" "ON L02-1"(w6485) -> ()
                  }
                }
              }
              frame #3 {
                n3663 = local read "SIG LAB02-2"() -> (w6489:T2)
                n3664 = Unbundle(w6489) -> ("AMPS"=w6488:dbl)  [unwired: 4 out]
                n3665 = Greater?(x=w6488, y=w6487) -> (0:w6486:bool)
                n3666 = case shown="True" w6486 {
                  frame False {
                  }
                  frame True {
                    n3667 = local read "ON L02-2"() -> (w6490:cluster{"amps":dbl, "volts":dbl, "pf":dbl})
                    n3668 = global write "Global display 2.vi" "ON L02-2"(w6490) -> ()
                  }
                }
              }
              frame #4 {
                n3669 = local read "SIG LAB03-1"() -> (w6494:T2)
                n3670 = Unbundle(w6494) -> ("AMPS"=w6493:dbl)  [unwired: 4 out]
                n3671 = Greater?(x=w6493, y=w6492) -> (0:w6491:bool)
                n3672 = case shown="True" w6491 {
                  frame False {
                  }
                  frame True {
                    n3673 = local read "ON L03-1"() -> (w6495:cluster{"amps":dbl, "volts":dbl, "pf":dbl})
                    n3674 = global write "Global display 2.vi" "ON L03-1"(w6495) -> ()
                  }
                }
              }
              frame #5 {
                n3675 = local read "SIG LAB03-2"() -> (w6499:T2)
                n3676 = Unbundle(w6499) -> ("AMPS"=w6498:dbl)  [unwired: 4 out]
                n3677 = Greater?(x=w6498, y=w6497) -> (0:w6496:bool)
                n3678 = case shown="True" w6496 {
                  frame False {
                  }
                  frame True {
                    n3679 = local read "ON L03-2"() -> (w6500:cluster{"amps":dbl, "volts":dbl, "pf":dbl})
                    n3680 = global write "Global display 2.vi" "ON L03-2"(w6500) -> ()
                  }
                }
              }
              frame #6 {
                n3681 = local read "SIG LAB04-1"() -> (w6504:T2)
                n3682 = Unbundle(w6504) -> ("AMPS"=w6503:dbl)  [unwired: 4 out]
                n3683 = Greater?(x=w6503, y=w6502) -> (0:w6501:bool)
                n3684 = case shown="True" w6501 {
                  frame False {
                  }
                  frame True {
                    n3685 = local read "ON L04-1"() -> (w6505:cluster{"amps":dbl, "volts":dbl, "pf":dbl})
                    n3686 = global write "Global display 2.vi" "ON L04-1"(w6505) -> ()
                  }
                }
              }
              frame #7 {
                n3687 = local read "SIG LAB04-2"() -> (w6509:T2)
                n3688 = Unbundle(w6509) -> ("AMPS"=w6508:dbl)  [unwired: 4 out]
                n3689 = Greater?(x=w6508, y=w6507) -> (0:w6506:bool)
                n3690 = case shown="True" w6506 {
                  frame False {
                  }
                  frame True {
                    n3691 = local read "ON L04-2"() -> (w6510:cluster{"amps":dbl, "volts":dbl, "pf":dbl})
                    n3692 = global write "Global display 2.vi" "ON L04-2"(w6510) -> ()
                  }
                }
              }
              frame #8 {
                n3693 = local read "SIG LAB05-1"() -> (w6514:T2)
                n3694 = Unbundle(w6514) -> ("AMPS"=w6513:dbl)  [unwired: 4 out]
                n3695 = Greater?(x=w6513, y=w6512) -> (0:w6511:bool)
                n3696 = case shown="True" w6511 {
                  frame False {
                  }
                  frame True {
                    n3697 = local read "ON L05-1"() -> (w6515:cluster{"amps":dbl, "volts":dbl, "pf":dbl})
                    n3698 = global write "Global display 2.vi" "ON L05-1"(w6515) -> ()
                  }
                }
              }
              frame #9 {
                n3699 = local read "SIG LAB05-2"() -> (w6519:T2)
                n3700 = Unbundle(w6519) -> ("AMPS"=w6518:dbl)  [unwired: 4 out]
